vi "CPP_Puff_release3_chs.vi"() -> (5 "Plug in titles":string[](array[string]), 7 "Plug in values":string[](array[string]))   [LabVIEW 2010]
uses:
  Controls/Post_Process.ctl
  Globals/Plug_in_data_global.vi
  Globals/Meas_global.vi
  <vilib>/measure/mascope.llb/Transition Measurements 1 chan.vi
  Globals/Dynamic_call_global.ph.vi
  <vilib>/measure/NI_MAPro.lvlib
panel:
  out "FFID1 2":cluster{dbl, dbl, dbl[]}[](graph)
  out "Valve":cluster{dbl, dbl, dbl[]}(graph)
  in  "Averaging Samples":i32=1 min=1
  out "ValveShutAt":dbl format="%.2f"
  out "FFID2":cluster{dbl, dbl, dbl[]}(graph)
  out "Current Block No":i32
  out "FFID1":cluster{dbl, dbl, dbl[]}(graph)
  out "SourceOffIndex":i32
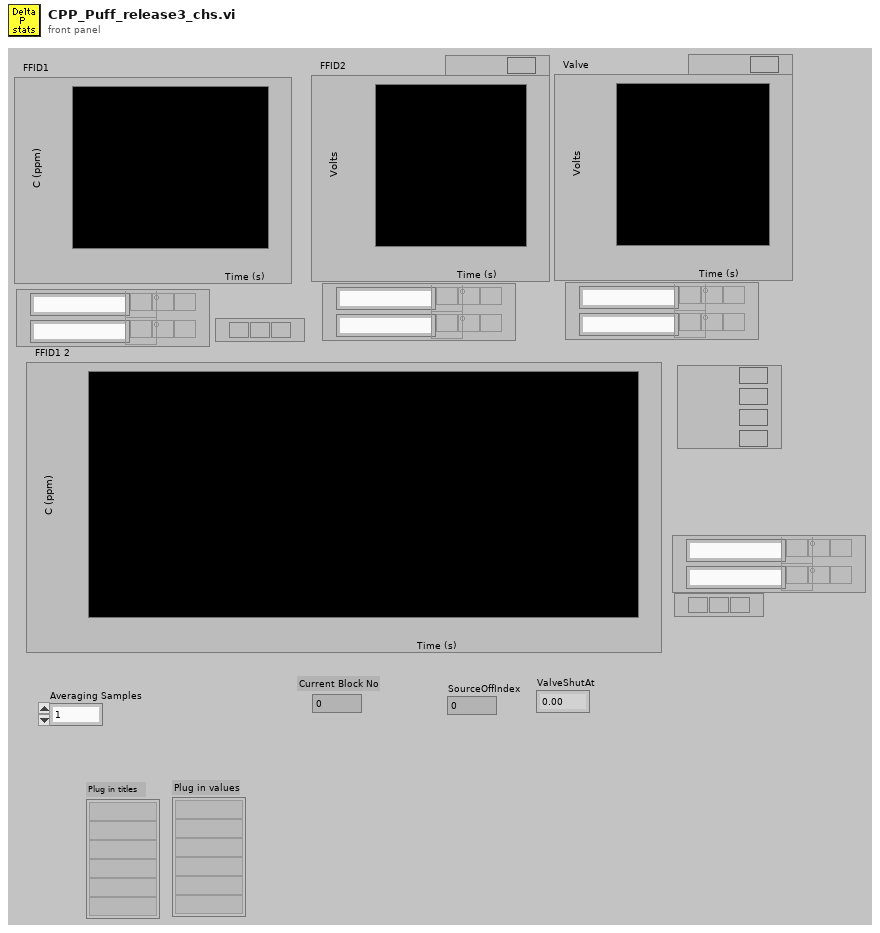
[diagram p1: front panel]
types:
  T1 = enum16{"Save no data", "Save data in new files", "Save data in existing files"}
  T2 = typedef "Post_Process.ctl" = enum16{"Take New Data", "Post Process Raw Data File"}
  T3 = cluster{"start time":dbl, "end time":dbl, "ref levels":cluster{"high ref level":dbl, "mid ref level":dbl, "low ref level":dbl, "ref units":u16}}
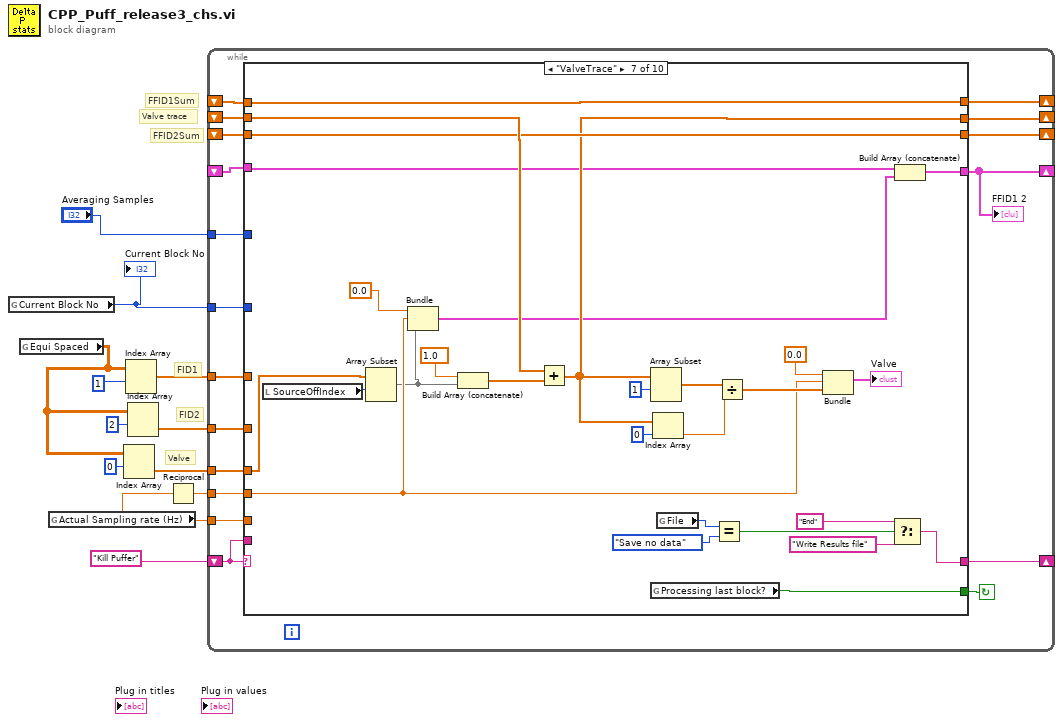
[diagram p0: block diagram]
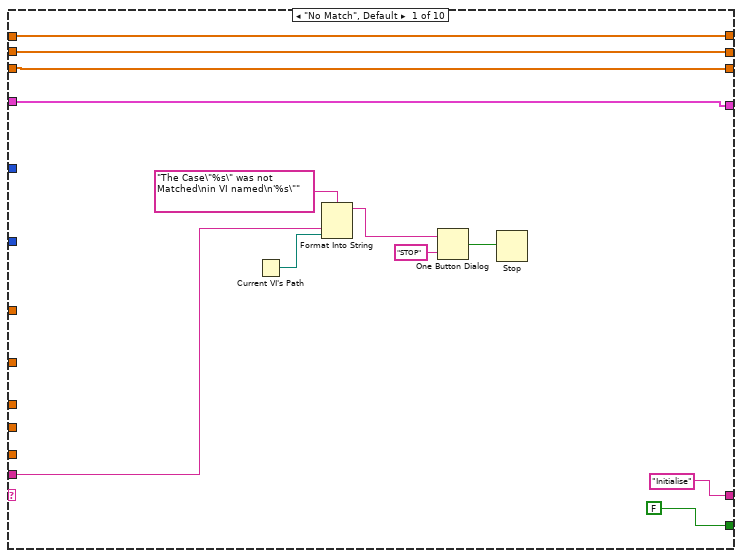
[diagram p2: hidden frame]
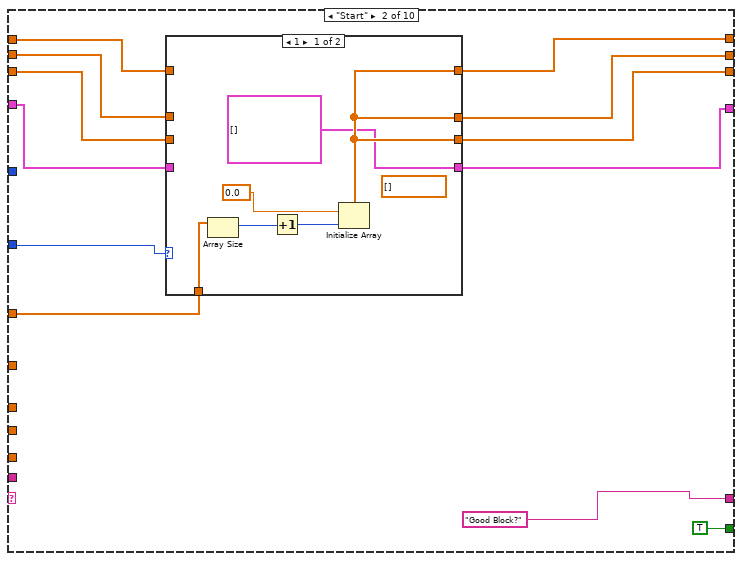
[diagram p3: hidden frame]
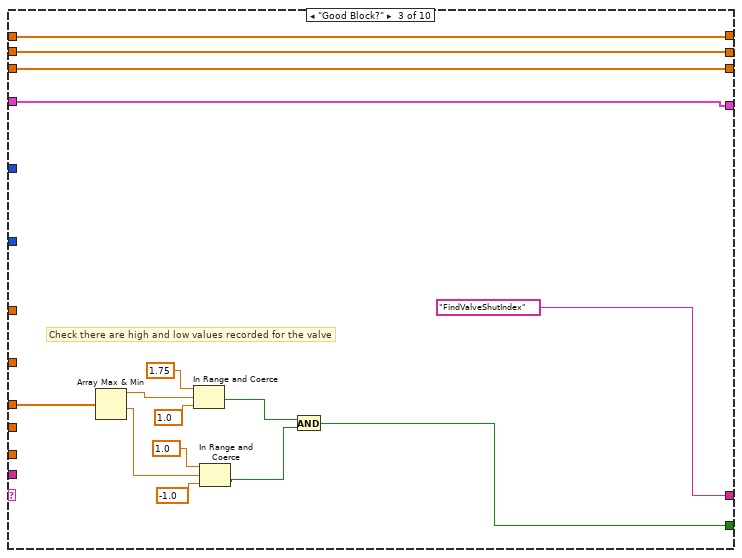
[diagram p5: hidden frame]
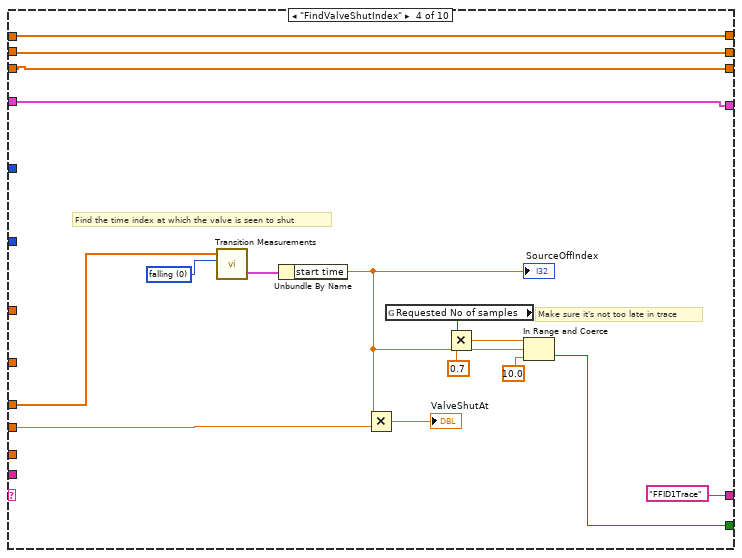
[diagram p6: hidden frame]
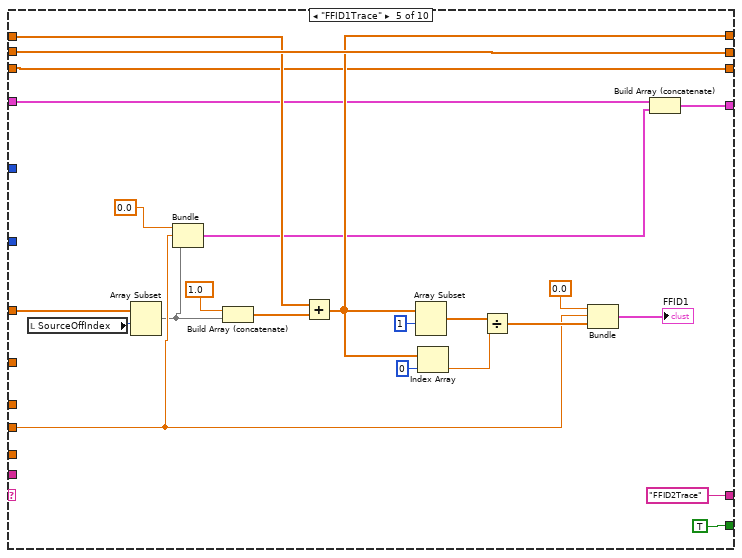
[diagram p7: hidden frame]
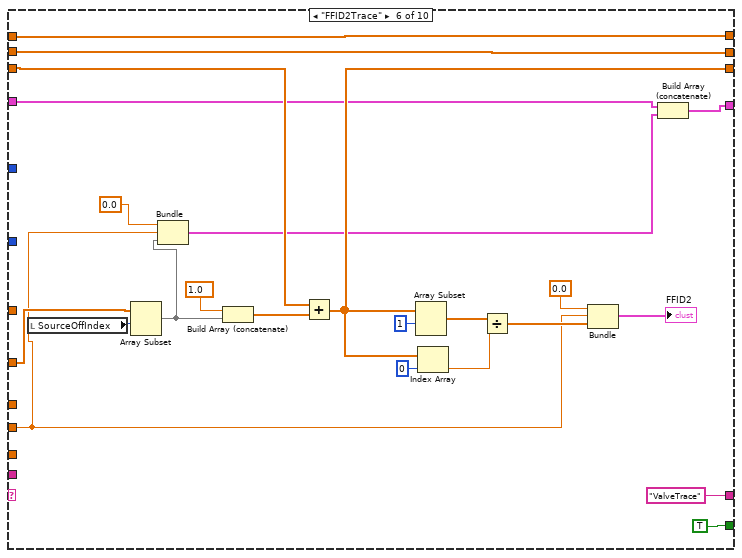
[diagram p8: hidden frame]
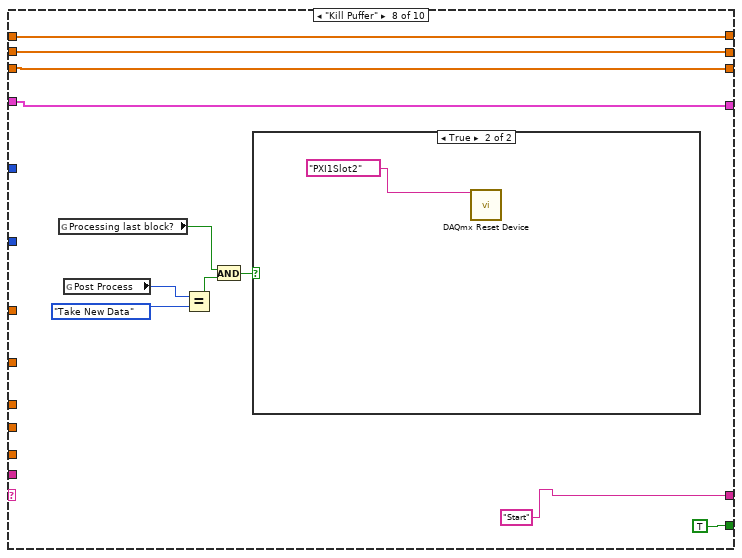
[diagram p9: hidden frame]
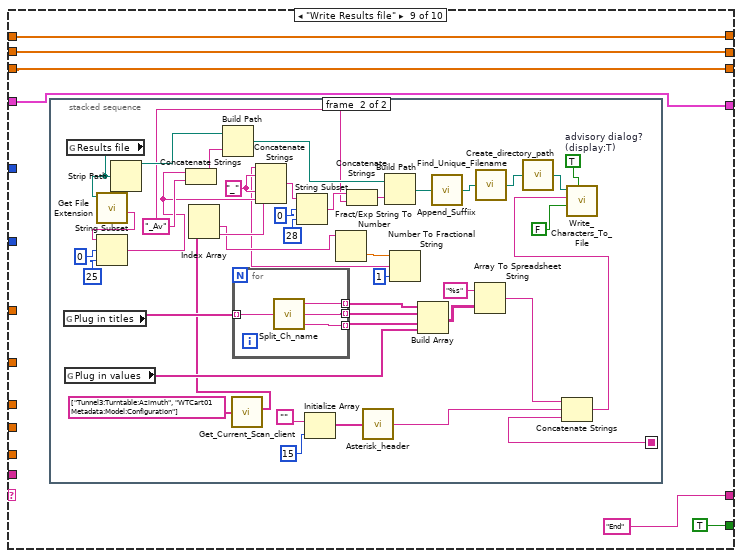
[diagram p11: hidden frame]
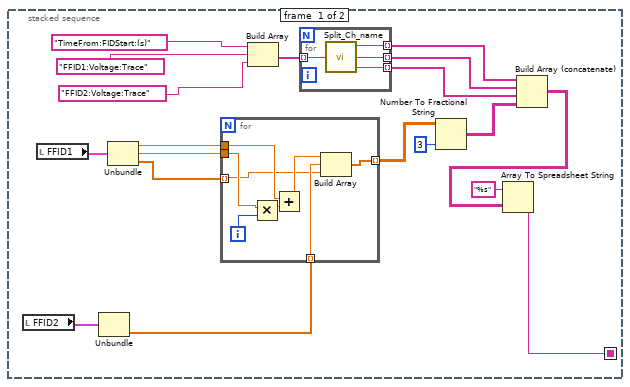
[diagram p12: hidden frame]
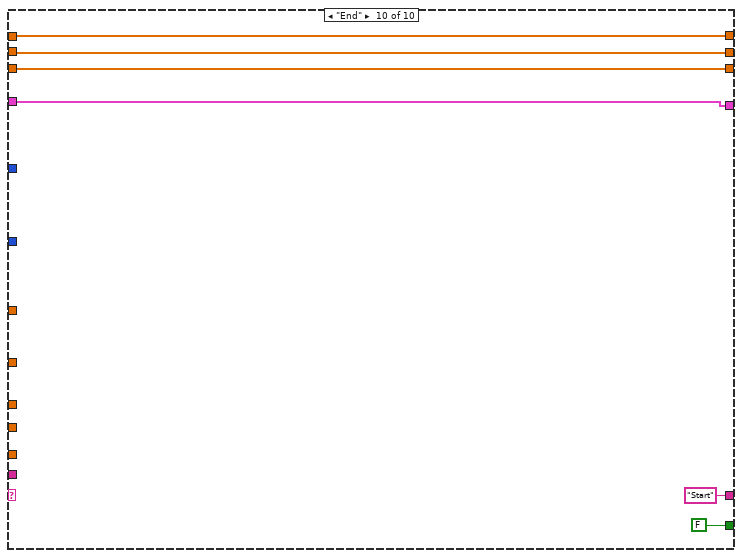
[diagram p13: hidden frame]
diagram:
  # "Valve"
  # "FID2"
  # "FID1"
  # "FFID2Sum"
  # "Valve trace"
  # "FFID1Sum"
  n1 = global read "Meas_global.vi" "Current Block No"() -> (w9:i32)
  "Current Block No" <- w9
  n2 = global read "Plug_in_data_global.vi" "Equi Spaced"() -> (w6:dbl[][])
  n3 = global read "Meas_global.vi" "Actual Sampling rate (Hz)"() -> (w2:dbl)
  n4 = Index Array(array=w6, index (row)=0) -> (element=w5:dbl[])  [unwired: 1 in]
  n5 = Index Array(array=w6, index (row)=1) -> (element=w10:dbl[])  [unwired: 1 in]
  n6 = Index Array(array=w6, index (row)=2) -> (element=w11:dbl[])  [unwired: 1 in]
  n7 = Reciprocal(x=w2) -> (1/x=w1:dbl)
  n8 = while {
    shift-left: "Kill Puffer" -> [w28]
    shift-right: [w29] -> _
    shift-right: [w27] -> _
    shift-left: _ -> [w24]
    shift-right: [w26] -> _
    shift-left: _ -> [w25]
    tunnel: w11 -> [w23]
    tunnel: w10 -> [w22]
    tunnel: w2 -> [w21]
    tunnel: w9 -> [w20]
    shift-right: [w18] -> _
    shift-left: _ -> [w17]
    tunnel: w5 -> [w19]
    tunnel: "Averaging Samples" -> [w16]
    tunnel: w1 -> [w15]
    shift-right: [w13] -> _
    shift-left: _ -> [w14]
    stop <- w30 continue-if-true
    n9 = case shown="\"ValveTrace\"" w28 {
      tunnel: [FALSE TRUE ("Processing last block?") w74 w84 TRUE ("Processing last block?") TRUE ("Processing last block?") w148 TRUE ("Processing last block?") TRUE ("Processing last block?") FALSE ("Processing last block?")] -> w30
      tunnel: ["Initialise" "Good Block?" "FindValveShutIndex" "FFID1Trace" "FFID2Trace" "ValveTrace" w142 "Start" "End" "Start" ("f")] -> w29
      tunnel: w28 -> [w37 _ _ _ _ _ _ _ _ _]
      tunnel: [w34 w53 w79 w94 w106 w128 w160 w180 w187 w270] -> w27
      tunnel: [w33 w51 w78 w93 w116 w139 w157 w179 w186 w269] -> w26
      tunnel: w25 -> [w33 w50 w78 w93 w116 w139 w159 w179 w186 w269]
      tunnel: w24 -> [w34 w52 w79 w94 w114 w128 w160 w180 w187 w270]
      tunnel: w23 -> [_ _ _ _ _ w129 _ _ _ _]
      tunnel: w22 -> [_ w49 _ _ w115 _ _ _ _ _]
      tunnel: w21 -> [_ _ _ _ _ _ _ _ _ _]
      tunnel: w20 -> [_ w48 _ _ _ _ _ _ _ _]
      tunnel: w19 -> [_ _ w70 w89 _ _ w156 _ _ _]
      tunnel: [w32 w47 w71 w92 w103 w126 w158 w175 w183 w268] -> w18
      tunnel: w17 -> [w32 w46 w71 w92 w103 w127 w158 w175 w183 w268]
      tunnel: w16 -> [_ _ _ _ _ _ _ _ _ _]
      tunnel: w15 -> [_ _ _ w81 w98 w121 w151 _ _ _]
      tunnel: [w31 w44 w65 w80 w100 w125 w155 w171 w182 w265] -> w13
      tunnel: w14 -> [w31 w43 w65 w80 w101 w124 w154 w171 w182 w265]
      frame "No Match", Default {
        n10 = Current VI's Path() -> (path=w36:path)
        n11 = Format Into String(format string="The Case\"%s\" was not Matched\nin VI named\n'%s\"" ("Format String"), w37, w36) -> (resulting string=w40:string)  [unwired: 2 in, 1 out]
        n12 = One Button Dialog(message=w40, button name ("OK")="STOP") -> (true=w38:bool)
        n13 = Stop(stop? (T)=w38) -> ()
      }
      frame "Start" {
        n14 = case shown="1" w48 {
          tunnel: [w57 w64] -> w53
          tunnel: w52 -> [_ w64]
          tunnel: [w57 w63] -> w51
          tunnel: w50 -> [_ w63]
          tunnel: w49 -> [w60 _]
          tunnel: [w57 w62] -> w47
          tunnel: w46 -> [_ w62]
          tunnel: [cluster{dbl, dbl, dbl[]}[] [] w61] -> w44
          tunnel: w43 -> [_ w61]
          frame 1 {
            (unwired) dbl[] []
            n15 = Array Size(array=w60) -> (size(s)=w59:i32)
            n16 = Increment(x=w59) -> (x+1=w56:i32)
            n17 = Initialize Array(0.0 ("element"), w56) -> (w57:dbl[])
          }
          frame 2, Default {
          }
        }
      }
      frame "Good Block?" {
        # "Check there are high and low values recorded for the valve"
        n18 = Array Max & Min(array=w70) -> (max value=w73:dbl, min value=w67:dbl)  [unwired: 2 out]
        n19 = In Range and Coerce(upper limit=1.75, x=w73, lower limit=1.0 ("y")) -> (In Range?=w75:bool)  [unwired: 1 out]
        n20 = In Range and Coerce(upper limit=1.0, x=w67, lower limit=-1.0 ("y")) -> (In Range?=w66:bool)  [unwired: 1 out]
        n21 = And(x=w75, y=w66) -> (x .and. y?=w74:bool)
      }
      frame "FindValveShutIndex" {
        w91 = u16 0 items=["falling", "rising"] ("polarity (rising)")
        # "Make sure it's not too late in trace"
        # "Find the time index at which the valve is seen to shut"
        n22 = call-poly <vilib>:"Transition Measurements.vi"("polarity (rising)"=w91, "signal in"=w89) -> ("measurement info"=w90:T3)  [unwired: 4 in, 5 out]
        n23 = Unbundle By Name(w90) -> ("start time"=w83:dbl)
        "SourceOffIndex" <- w83
        n24 = Multiply(x=w83, y=w81) -> (x*y=→"ValveShutAt":dbl)
        n25 = global read "Meas_global.vi" "Requested No of samples"() -> (w88:i32)
        n26 = Multiply(x=w88, y=0.7 ("lower limit")) -> (x*y=w86:dbl)
        n27 = In Range and Coerce(upper limit=w86, x=w83, lower limit=10.0) -> (In Range?=w84:bool)  [unwired: 1 out]
      }
      frame "FFID1Trace" {
        n28 = local read "SourceOffIndex"() -> (w111:i32)
        n29 = Array Subset(array=w115, index=w111) -> (w97:dbl[])  [unwired: 1 in]
        n30 = Bundle(0.0, w98, w97) -> (w96:cluster{dbl, dbl, dbl[]})  [unwired: 1 out]
        n31 = Build Array (concatenate)(1.0, w97) -> (w112:dbl[])
        n32 = Add(x=w114, y=w112) -> (x+y=w106:dbl[])
        n33 = Array Subset(array=w106, index=1) -> (w105:dbl[])  [unwired: 1 in]
        n34 = Index Array(array=w106, index=0) -> (element=w104:dbl)
        n35 = Divide(x=w105, y=w104) -> (x/y=w110:dbl[])
        n36 = Bundle(0.0, w98, w110) -> (→"FFID1":cluster{dbl, dbl, dbl[]})  [unwired: 1 out]
        n37 = Build Array (concatenate)(w101, w96) -> (w100:cluster{dbl, dbl, dbl[]}[])
      }
      frame "FFID2Trace" {
        n38 = local read "SourceOffIndex"() -> (w136:i32)
        n39 = Array Subset(array=w129, index=w136) -> (w120:dbl[])  [unwired: 1 in]
        n40 = Bundle(0.0, w121, w120) -> (w119:cluster{dbl, dbl, dbl[]})  [unwired: 1 out]
        n41 = Build Array (concatenate)(1.0, w120) -> (w137:dbl[])
        n42 = Add(x=w127, y=w137) -> (x+y=w126:dbl[])
        n43 = Array Subset(array=w126, index=1) -> (w131:dbl[])  [unwired: 1 in]
        n44 = Index Array(array=w126, index=0) -> (element=w130:dbl)
        n45 = Divide(x=w131, y=w130) -> (x/y=w135:dbl[])
        n46 = Bundle(0.0, w121, w135) -> (→"FFID2":cluster{dbl, dbl, dbl[]})  [unwired: 1 out]
        n47 = Build Array (concatenate)(w124, w119) -> (w125:cluster{dbl, dbl, dbl[]}[])
      }
      frame "ValveTrace" {
        n48 = local read "SourceOffIndex"() -> (w167:i32)
        n49 = Array Subset(array=w156, index=w167) -> (w150:dbl[])  [unwired: 1 in]
        n50 = Bundle(0.0, w151, w150) -> (w149:cluster{dbl, dbl, dbl[]})  [unwired: 1 out]
        n51 = Build Array (concatenate)(1.0, w150) -> (w168:dbl[])
        n52 = Add(x=w159, y=w168) -> (x+y=w157:dbl[])
        n53 = Array Subset(array=w157, index=1) -> (w162:dbl[])  [unwired: 1 in]
        n54 = global read "Meas_global.vi" "Processing last block?"() -> (w148:bool)
        n55 = Index Array(array=w157, index=0) -> (element=w161:dbl)
        n56 = global read "Meas_global.vi" "File"() -> (w147:T1)
        n57 = Equal?(x=w147, y=T1."Save no data" ("File")) -> (x = y?=w143:bool)
        n58 = Divide(x=w162, y=w161) -> (x/y=w166:dbl[])
        n59 = Bundle(0.0, w151, w166) -> (→"Valve":cluster{dbl, dbl, dbl[]})  [unwired: 1 out]
        n60 = Select(t="End", s=w143, f="Write Results file") -> (s? t:f=w142:string)
        n61 = Build Array (concatenate)(w154, w149) -> (w155:cluster{dbl, dbl, dbl[]}[])
      }
      frame "Kill Puffer" {
        n62 = global read "Meas_global.vi" "Processing last block?"() -> (w174:bool)
        n63 = global read "Meas_global.vi" "Post Process"() -> (w177:T2)
        n64 = Equal?(x=w177, y=Post_Process."Take New Data" ("Post Process")) -> (x = y?=w173:bool)
        n65 = And(x=w174, y=w173) -> (x .and. y?=w172:bool)
        n66 = case shown="True" w172 {
          frame False {
          }
          frame True {
            n67 = call <vilib>:"DAQmx Reset Device.vi"("device in"=tag "PXI1Slot2") -> ()  [unwired: 14 in, 1 out]
          }
        }
      }
      frame "Write Results file" {
        n68 = stacked-sequence {
          seq-local: [w196 _] -> [_ w246]
          frame #0 {
            n69 = local read "FFID2"() -> (w195:cluster{dbl, dbl, dbl[]})
            n70 = local read "FFID1"() -> (w206:cluster{dbl, dbl, dbl[]})
            n71 = Unbundle(w195) -> (w194:dbl[])  [unwired: 2 out]
            n72 = Unbundle(w206) -> (w204:dbl, w205:dbl, w203:dbl[])
            n73 = for {
              tunnel: w205 -> [w217]
              tunnel: w204 -> [w216]
              tunnel: w203 -> [w211] mode=indexing
              tunnel: [w214] -> w201 mode=indexing
              tunnel: w194 -> [w212] mode=indexing
              i -> [w218]
              n74 = Multiply(x=w217, y=w218) -> (x*y=w215:dbl)
              n75 = Add(x=w216, y=w215) -> (x+y=w213:dbl)
              n76 = Build Array(w213, w212, w211) -> (w214:dbl[])
            }
            n77 = Build Array("TimeFrom:FIDStart:(s)", "FFID1:Voltage:Trace", "FFID2:Voltage:Trace") -> (w191:string[])
            n78 = for {
              tunnel: w191 -> [w210] mode=indexing
              tunnel: [w209] -> w190 mode=indexing
              tunnel: [w208] -> w189 mode=indexing
              tunnel: [w207] -> w188 mode=indexing
              n79 = call "Split_Ch_name.vi"("Ch name"=w210) -> ("Top level"=w209:string, "Middle"=w208:string, "Low level"=w207:string)
            }
            n80 = Number To Fractional String(number=w201, precision (6)=i16 3) -> (F-format string=w200:string[][])  [unwired: 2 out]
            n81 = Build Array (concatenate)(w190, w189, w188, w200) -> (w198:string[][])
            n82 = Array To Spreadsheet String(array=w198, 3:"%s" ("format string")) -> (spreadsheet string=w196:string)  [unwired: 1 out]
          }
          frame #1 {
            w234 = "_" ("string")
            w260 = TRUE  # advisory dialog? (display:T)
            w230 = "_Av" ("string")
            n83 = global read "Dynamic_call_global.ph.vi" "Plug in titles"() -> (w258:string[])
            n84 = global read "Dynamic_call_global.ph.vi" "Plug in values"() -> (w254:string[])
            n85 = global read "Meas_global.vi" "Results file"() -> (w240:path)
            n86 = call <vilib>:"Get File Extension.vi"("file"=w240) -> ("filename without extension"=w226:string)  [unwired: 7 in, 3 out]
            n87 = String Subset(string=w226, offset (0)=0, length (rest)=25 ("length (rest)")) -> (substring=w225:string)
            n88 = Strip Path(path=w240) -> (stripped path=w239:path)  [unwired: 1 out]
            n89 = Concatenate Strings(w225, w230) -> (w237:string)
            n90 = Build Path(base path=w239, name or relative path=w237) -> (appended path=w238:path)
            n91 = call "Get_Current_Scan_client.vi"("ADAM Ch Names"=string[] ["Tunnel3:Turntable:Azimuth", "WTCart01 Metadata:Model:Configuration"]) -> ("String values"=w235:string[])  [unwired: 1 in, 2 out]
            n92 = Index Array(array=w235) -> (element #1=w222:string, element #2=w233:string)  [unwired: 2 in]
            n93 = for {
              tunnel: w258 -> [w264] mode=indexing
              tunnel: [w263] -> w257 mode=indexing
              tunnel: [w262] -> w256 mode=indexing
              tunnel: [w261] -> w255 mode=indexing
              n94 = call "Split_Ch_name.vi"("Ch name"=w264) -> ("Top level"=w263:string, "Middle"=w262:string, "Low level"=w261:string)
            }
            n95 = Initialize Array("", 15) -> (w251:string[])
            n96 = Fract/Exp String To Number(string=w222) -> (number=w221:dbl)  [unwired: 3 in, 1 out]
            n97 = call "Asterisk_header.vi"("Channel names"=w251) -> ("Header string"=w247:string)
            n98 = Number To Fractional String(number=w221, precision (6)=i16 1) -> (F-format string=w219:string)  [unwired: 2 in]
            n99 = Concatenate Strings(w219, w234, w233, w234, w225) -> (w232:string)
            n100 = String Subset(string=w232, offset (0)=0, length (rest)=28 ("length (rest)")) -> (substring=w231:string)
            n101 = Concatenate Strings(w231, w230) -> (w229:string)
            n102 = Build Path(base path=w238, name or relative path=w229) -> (appended path=w242:path)
            n103 = Build Array(w257, w256, w255, w254) -> (w252:string[][])
            n104 = call "Append_Suffiix.vi"("Results file"=w242) -> ("appended path"=w241:path)
            n105 = Array To Spreadsheet String(array=w252, 3:"%s" ("format string")) -> (spreadsheet string=w248:string)  [unwired: 1 out]
            n106 = call "Find_Unique_Filename.vi"("Path In"=w241) -> ("Unique Path Out"=w224:path)  [unwired: 1 in, 1 out]
            n107 = call "Create_directory_path.vi"("Path name"=w224) -> ("Path name Out"=w223:path)
            n108 = Concatenate Strings(w248, w247, w246) -> (w245:string)
            n109 = call "Write_Characters_To_File.vi"("file path (dialog if empty)"=w223, "advisory dialog? (display:T)"=w260, "character string"=w245, "append to file? (new file:F)"=FALSE) -> ()  [unwired: 1 in, 4 out]
          }
        }
      }
      frame "End" {
      }
    }
    "FFID1 2" <- w13
  }
